vi "Lab2.vi"() -> ()   [LabVIEW 2021]
panel:
  out "recieved string":string
  in  "string":string
  out "bytes written":i32
  in  "sendbutton":bool
  in  "stop":bool
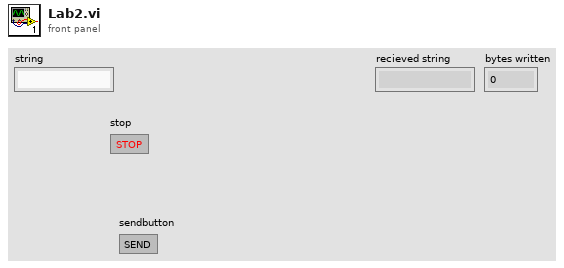
[diagram p1: front panel]
types:
  T1 = enum16{"Standard", "Buffered", "CRLF", "Immediate"}
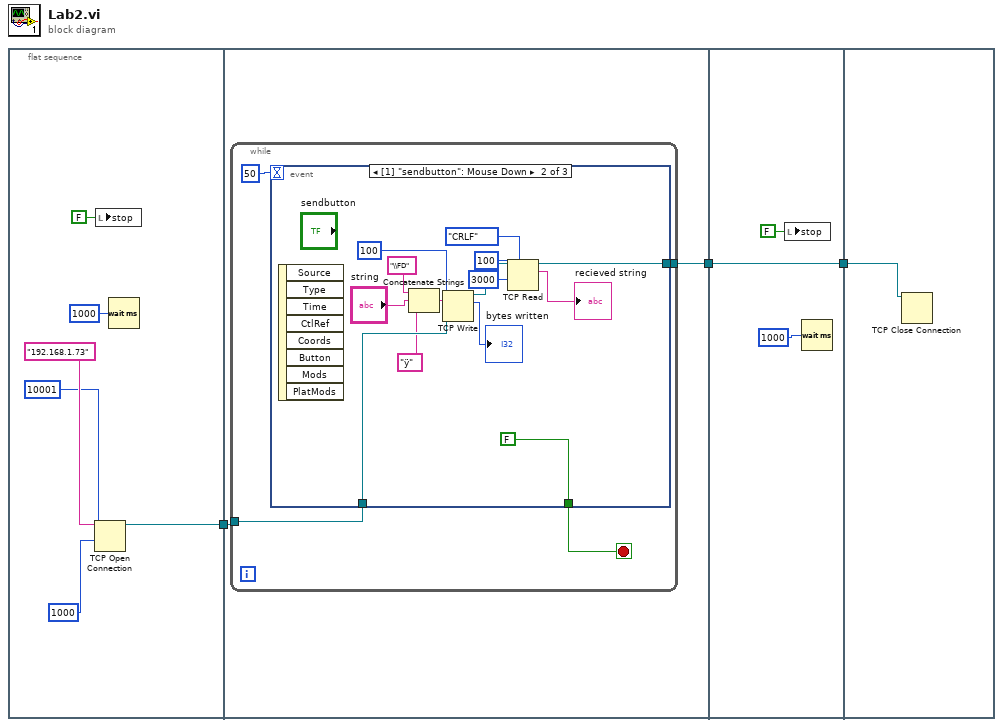
[diagram p0: block diagram]
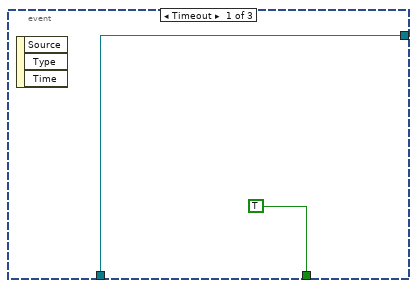
[diagram p2: hidden frame]
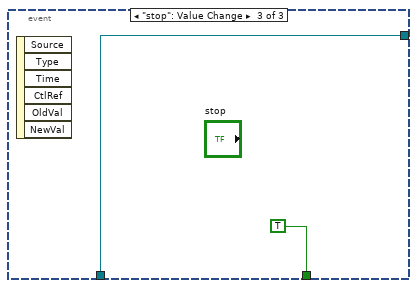
[diagram p3: hidden frame]
diagram:
  n1 = flat-sequence {
    tunnel: [w4] -> w3
    tunnel: w3 -> [w11]
    tunnel: [w10] -> w1
    tunnel: [w34] -> w2
    tunnel: w1 -> [w34]
    tunnel: w2 -> [w37]
    frame #0 {
      n2 = TCP Open Connection(address="192.168.1.73", remote port or service name=u16 10001, timeout ms (60000)=1000) -> (connection ID=w4:refnum<k5>)  [unwired: 2 in, 1 out]
      n3 = local write "stop"(FALSE ("stop")) -> ()
      n4 = Wait (ms)(milliseconds to wait=u32 1000) -> ()  [unwired: 1 out]
    }
    frame #1 {
      n5 = while {
        tunnel: w11 -> [w15]
        tunnel: [w14] -> w10
        stop <- w12 stop-if-true
        n6 = event shown="[1] \"sendbutton\": Mouse Down" {
          selector: _ -> [_ _ _]
          dyn-events: _ -> [_ _ _]
          timeout: 50 -> [_ _ _]
          tunnel: w15 -> [w17 w31 w33]
          tunnel: [w17 w23 w33] -> w14
          tunnel: [TRUE FALSE ("stop") TRUE] -> w12
          event Timeout {
            n7 = event-data() -> ()  [unwired: 1 in, 3 out]
          }
          event "sendbutton": Mouse Down {
            n8 = event-data() -> ()  [unwired: 1 in, 8 out]
            n9 = Concatenate Strings("\\FD" ("string"), "string", "ÿ" ("string")) -> (w29:string)
            n10 = TCP Write(connection ID=w31, data in=w29, 9:100 ("timeout ms (25000)")) -> (connection ID out=w24:refnum<k5>, bytes written=→"bytes written":i32)  [unwired: 1 in, 1 out]
            n11 = TCP Read(connection ID=w24, bytes to read=100, 7:T1."CRLF" ("mode (standard)"), 9:3000 ("timeout ms (25000)")) -> (connection ID out=w23:refnum<k5>, data out=→"recieved string":string)  [unwired: 1 in, 1 out]
          }
          event "stop": Value Change {
            n12 = event-data() -> ()  [unwired: 1 in, 6 out]
          }
        }
      }
    }
    frame #2 {
      n13 = local write "stop"(FALSE ("stop")) -> ()
      n14 = Wait (ms)(milliseconds to wait=u32 1000) -> ()  [unwired: 1 out]
    }
    frame #3 {
      n15 = TCP Close Connection(connection ID=w37) -> ()  [unwired: 2 in, 2 out]
    }
  }
